vi "EscapeJsonString.vi"(8 "error in (no error)":errorcluster, 11 "String in":string) -> (0 "error out":errorcluster, 3 "String out":string)   [LabVIEW 2017]
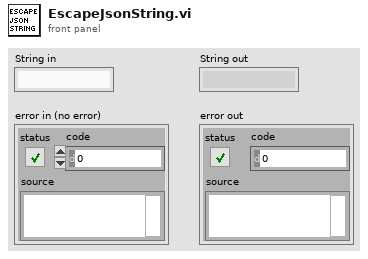
[diagram p1: front panel]
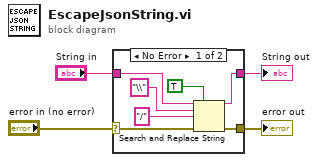
[diagram p0: block diagram]
diagram:
  n1 = case shown="No Error" "error in (no error)" {
    selector: "error in (no error)" -> [w11 w13]
    tunnel: [w10 w12] -> w3
    tunnel: [w9 w13] -> w2
    tunnel: "String in" -> [w8 w12]
    frame No Error {
      n2 = Search and Replace String(replace all?=TRUE ("replace all? (F)"), input string=w8, search string="\\", replace string="/" ("search string"), error in=w11) -> (result string=w10:string, error out=w9:errorcluster)  [unwired: 3 in, 2 out]
    }
    frame Error {
    }
  }
  "String out" <- w3
  "error out" <- w2
